vi "Generate Unique Header.vi"(8 "error in":errorcluster, 11 "PAS Data in":refnum<class "PAS Data.lvclass">) -> (0 "error out":errorcluster, 2 "Header":string[](array[string]), 3 "PAS Data out":refnum<class "PAS Data.lvclass">)   [LabVIEW 2014, in "PAS Library.lvlib" / "PAS Data.lvclass"]
uses:
  PAS Data.lvclass
  Data/Data.lvclass/Data.ctl
  PAS Data.lvclass/PAS Data.ctl
  Data/Read Data ID.vi
  Cell/PAS Cell Data.lvclass
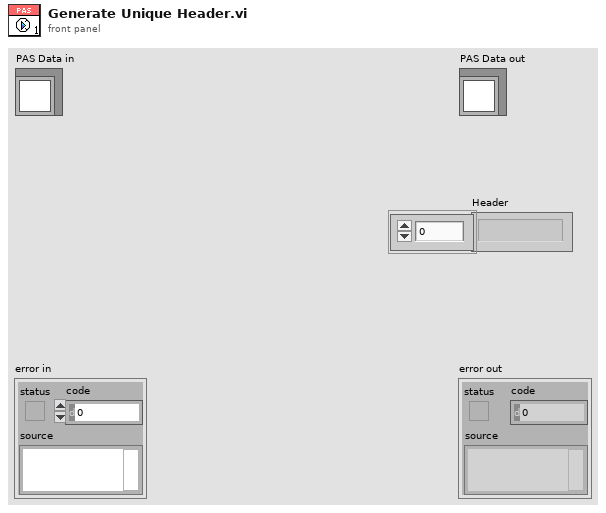
[diagram p1: front panel]
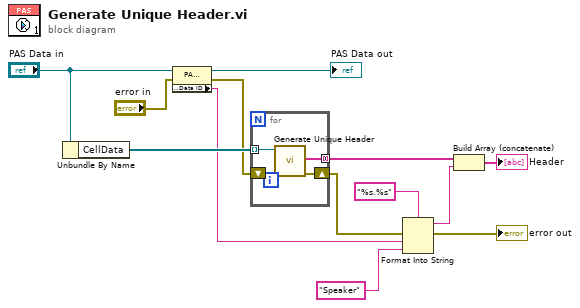
[diagram p0: block diagram]
diagram:
  n1 = Unbundle By Name("PAS Data in") -> ("CellData"=w13:refnum<class "PAS Cell Data.lvclass">[])
  n2 = property class="PAS Data"(reference="PAS Data in", error in="error in") -> (reference out=→"PAS Data out":refnum<class "PAS Data.lvclass">, error out=w3:errorcluster, "Accessors:Data ID"=w7:string)
  n3 = for {
    tunnel: w13 -> [w17] mode=indexing
    tunnel: [w16] -> w12 mode=concatenating
    shift-right: [w14] -> w2
    shift-left: w3 -> [w15]
    n4 = call-dynamic "Generate Unique Header.vi"("error in"=w15, "PAS Cell Data in"=w17) -> ("error out"=w14:errorcluster, "Header"=w16:string[])  [unwired: 7 in, 1 out]
  }
  n5 = Format Into String(format string="%s.%s", error in=w2, w7, "Speaker") -> (resulting string=w5:string, error out=→"error out":errorcluster)  [unwired: 1 in]
  n6 = Build Array (concatenate)(w12, w5) -> (→"Header":string[])
